vi "BuildServer INI Tool.vi"(7 "WorkerShow":bool=TRUE, 8 "error in (no error)":errorcluster, 9 "CommPort":u32=4545, 10 "WorkerFolder":path=path "/Volumes/Data/Users/benji667/Git/BuildFarm/src/BuildWorker", 11 "WorkerInterface":string="BuildWorker Basics.lvclass") -> (0 "error out":errorcluster, 3 "file path":path)   [LabVIEW 2017]
uses:
  <vilib>/Utility/config.llb/Write Key (String).vi
  <vilib>/Utility/config.llb/Write Key (Path).vi
  <vilib>/Utility/config.llb/Write Key (Boolean).vi
  <vilib>/Utility/config.llb/Write Key (U32).vi
  <vilib>/Utility/config.llb/NI_LVConfig.lvlib
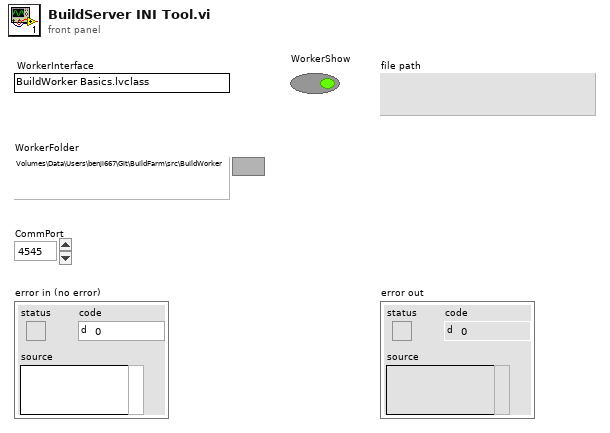
[diagram p1: front panel]
types:
  T1 = typedef "NI_LVConfig.lvlib/Config Data RefNum.ctl" = refnum<k1>
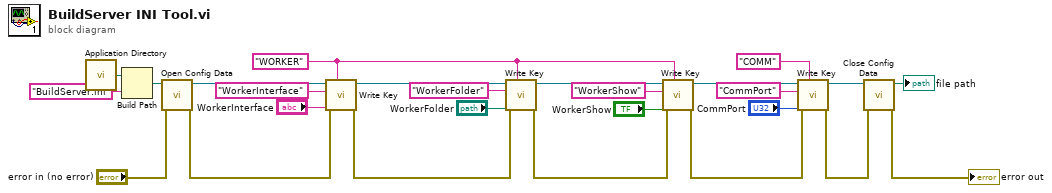
[diagram p0: block diagram]
diagram:
  w7 = "WORKER" ("section")
  n1 = call <vilib>:"Application Directory.vi"() -> ("Application Directory"=w26:path)
  n2 = Build Path(base path=w26, name or relative path="BuildServer.ini") -> (appended path=w6:path)
  n3 = call <vilib>:"Open Config Data.vi"("error in (no error)"="error in (no error)", "configuration file path"=w6) -> ("error out"=w23:errorcluster, "refnum"=w24:T1)  [unwired: 7 in, 1 out]
  n4 = call-poly <vilib>:"Write Key.vi"("section"=w7, "error in (no error)"=w23, "value"="WorkerInterface", "key"="WorkerInterface", "refnum"=w24) -> ("error out"=w9:errorcluster, "refnum out"=w12:T1)  [unwired: 4 in, 1 out]
  n5 = call-poly <vilib>:"Write Key.vi"("section"=w7, "error in (no error)"=w9, "value"="WorkerFolder", "key"="WorkerFolder", "refnum"=w12) -> ("error out"=w8:errorcluster, "refnum out"=w11:T1)  [unwired: 4 in, 1 out]
  n6 = call-poly <vilib>:"Write Key.vi"("section"=w7, "error in (no error)"=w8, "value"="WorkerShow", "key"="WorkerShow", "refnum"=w11) -> ("error out"=w17:errorcluster, "refnum out"=w18:T1)  [unwired: 4 in, 1 out]
  n7 = call-poly <vilib>:"Write Key.vi"("section"="COMM", "error in (no error)"=w17, "value"="CommPort", "key"="CommPort", "refnum"=w18) -> ("error out"=w15:errorcluster, "refnum out"=w16:T1)  [unwired: 4 in, 1 out]
  n8 = call <vilib>:"Close Config Data.vi"("error in (no error)"=w15, "refnum"=w16) -> ("error out"=→"error out":errorcluster, "file path"=→"file path":path)  [unwired: 8 in]
